vi "rpr -- read segment files.vi"(0 "9w folder path":path=path "C:/data/RUS/Experiment/ProbeTest/Probe10/YBCO_5/sweep2/9w", 2 "segment index":i32=2, 5 "buttons":bool[](array[boolean])=[TRUE, TRUE, TRUE, TRUE, TRUE, TRUE, TRUE, TRUE, TRUE, TRUE, TRUE, TRUE, TRUE, TRUE, TRUE, TRUE, TRUE, TRUE, TRUE, TRUE, TRUE, TRUE, TRUE, TRUE, TRUE, TRUE, TRUE, TRUE, TRUE], 6 "what":T2(ring)=enum."norm. attenuation", 8 "averaging window":i32=5, 10 "min T":dbl=nan, 12 "max T":dbl=nan) -> (9 "# of peaks":i32, 11 "# of temperatures":i32, 13 "K per min":dbl, 14 "peaks":i32[](array[numeric]), 16 "temperature points OUT":dbl[](array[numeric]), 17 "all peaks":i32[](array[numeric]), 18 "all unfiltered":T3(array[cluster]), 19 "Array":dbl[][](array[numeric]))   [LabVIEW 2014]
uses:
  segment file kind.ctl
  tale of three indices.vi
  Q -- check range -- i -- integer.vi
  linear interpolation - real.vi
  line -- complex.vi
  <vilib>/Analysis/baseanly.llb/A x B.vi
  <vilib>/Analysis/baseanly.llb/Real A x B.vi
  Q -- check range -- i -- real.vi
  command stack.vi
  tale of three indices -- check state.vi
  Q - not nan -- integer.vi
  Q - not nan -- real.vi
  <vilib>/Utility/file.llb/Read From Spreadsheet File.vi
  <vilib>/Utility/file.llb/Read From Spreadsheet File (string).vi
  <vilib>/Analysis/Matrix/Numeric/Conversions/Array To Matrix.vi
  <vilib>/Analysis/Matrix/Numeric/Conversions/Array To Matrix - RA2.vi
  <vilib>/Analysis/baseanly.llb/Inverse Matrix.vi
  <vilib>/Analysis/baseanly.llb/Real Inverse Matrix.vi
  <vilib>/regexp/Match Regular Expression.xnode
  <vilib>/Analysis/NI_AALBase.lvlib
panel:
  in  "segment file kind":T1
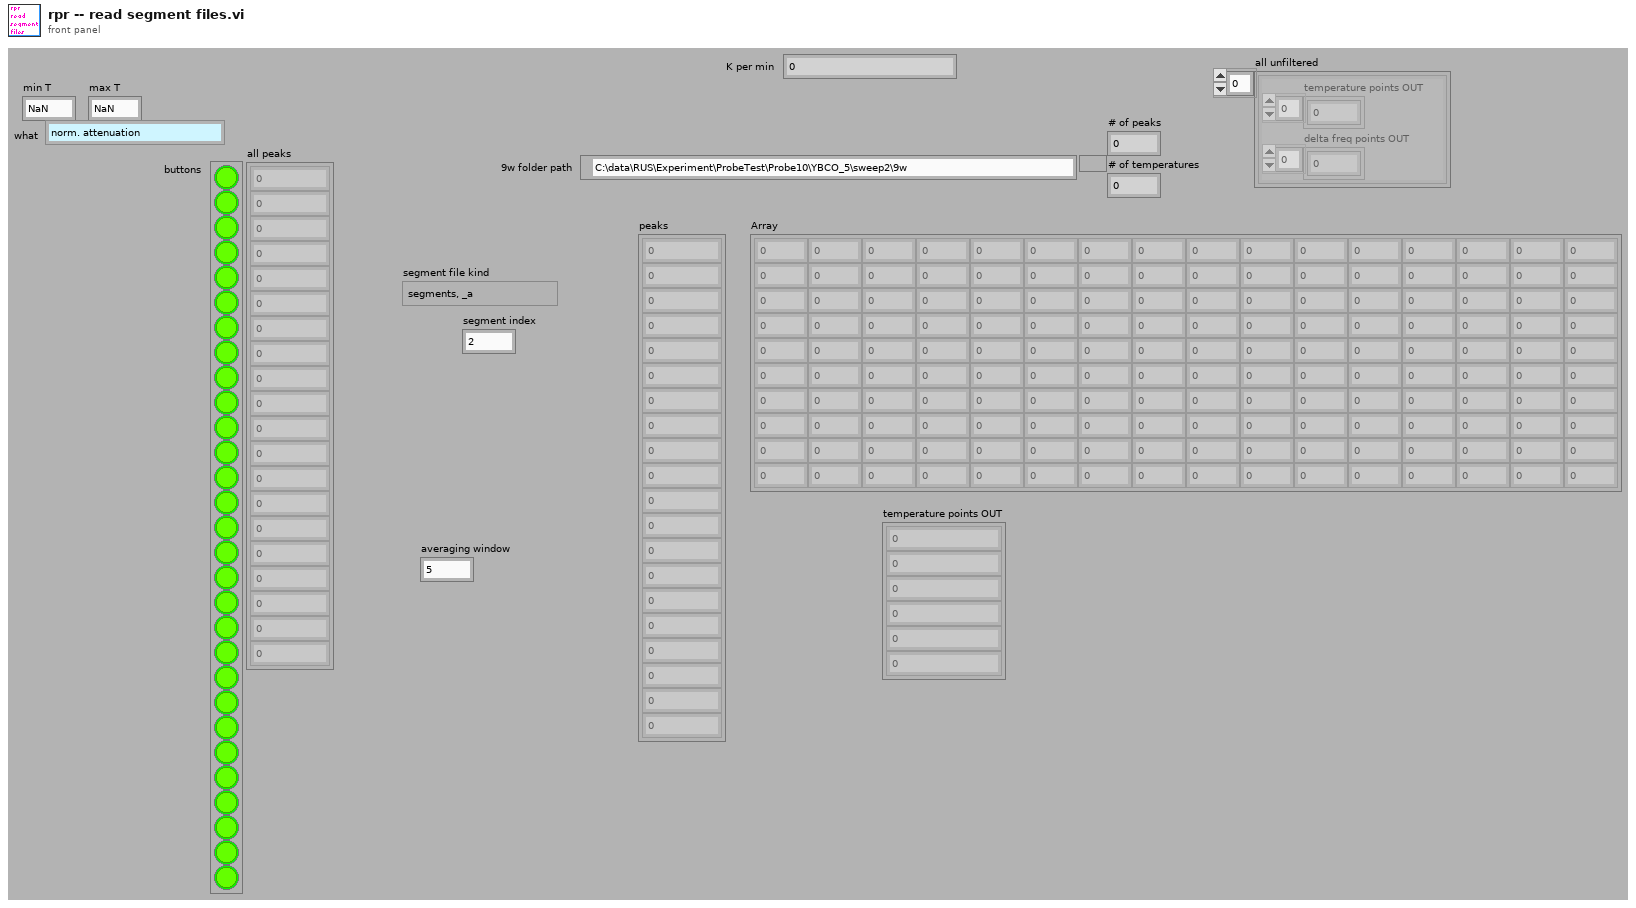
[diagram p1: front panel]
types:
  T1 = typedef "segment file kind.ctl" = enum16{"segments, _a", "monitor, _m", "other"}
  T2 = enum16{"frequency", "attenuation", "deltafreq", "Vardeltafreq", "log 1/Q", "1/Q", "norm. attenuation", "log gamma", "VarDeltaFreq div f"}
  T3 = cluster{"temperature points OUT":dbl[], "delta freq points OUT":dbl[]}[]
  T4 = cluster{"temperature points OUT":dbl[], "z out":dbl[]}
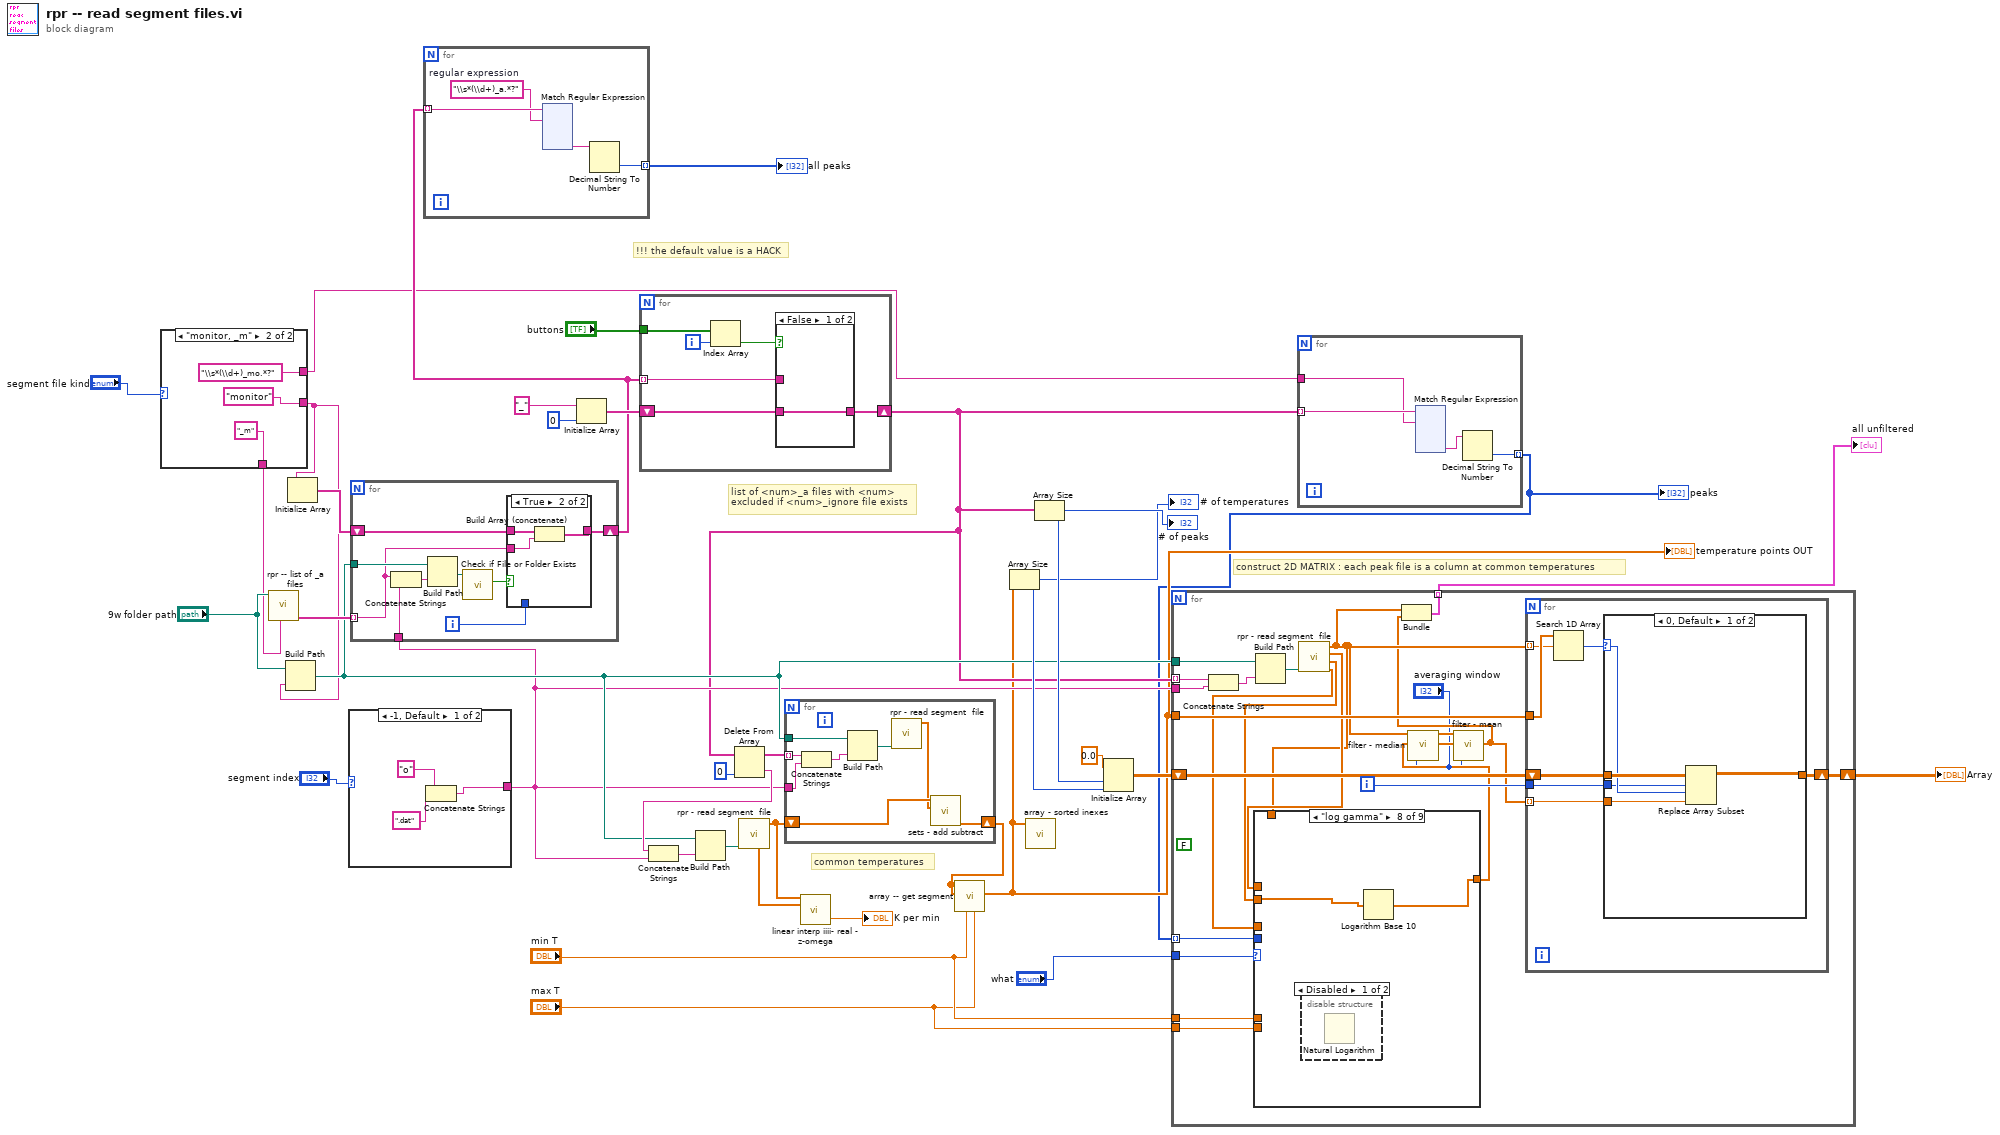
[diagram p0: block diagram]
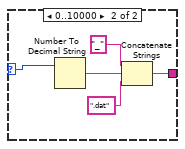
[diagram p2: hidden frame]
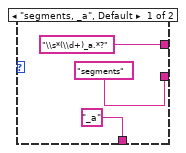
[diagram p3: hidden frame]
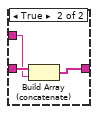
[diagram p4: hidden frame]
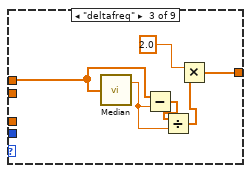
[diagram p8: hidden frame]
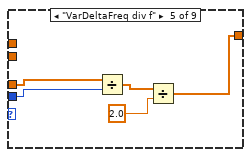
[diagram p10: hidden frame]
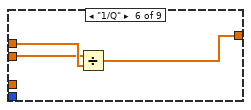
[diagram p11: hidden frame]
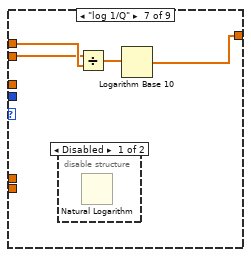
[diagram p12: hidden frame]
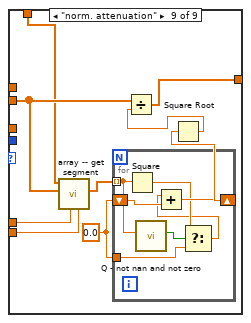
[diagram p15: hidden frame]
diagram:
  # "!!! the default value is a HACK"
  # "list of <num>_a files with <num> \nexcluded if <num>_ignore file exists"
  # "construct 2D MATRIX : each peak file is a column at common temperatures"
  # "common temperatures"
  n1 = case shown="\"monitor, _m\"" "segment file kind" {
    tunnel: ["segments" ("string") "monitor" ("string")] -> w7
    tunnel: ["_a" ("string") "_m" ("string")] -> w6
    tunnel: ["\\s*(\\d+)_a.*?" ("regular expression") "\\s*(\\d+)_mo.*?" ("regular expression")] -> w5
    frame "segments, _a", Default {
    }
    frame "monitor, _m" {
    }
  }
  n2 = call "rpr -- list of _a files.vi"("suffix"=w6, "9w folder path"="9w folder path") -> ("Array"=w28:string[])  [unwired: 9 in]
  n3 = Build Path(base path="9w folder path", name or relative path=w7) -> (appended path=w26:path)
  n4 = Initialize Array(w7) -> (w16:string[])  [unwired: 1 in]
  n5 = case shown="-1, Default" "segment index" {
    selector: "segment index" -> [_ w47]
    tunnel: [w45 w48] -> w25
    frame -1, Default {
      n6 = Concatenate Strings("o" ("string"), ".dat" ("string")) -> (w45:string)
    }
    frame 0..10000 {
      n7 = Number To Decimal String(number=w47) -> (decimal integer string=w51:string)  [unwired: 1 in]
      n8 = Concatenate Strings("_" ("string"), w51, ".dat" ("string")) -> (w48:string)
    }
  }
  n9 = for {
    tunnel: w26 -> [w59]
    tunnel: w28 -> [w52] mode=indexing
    tunnel: w25 -> [w58]
    shift-right: [w55] -> w18
    shift-left: w16 -> [w56]
    i -> [w54]
    n10 = Concatenate Strings(w52, w58) -> (w60:string)
    n11 = Build Path(base path=w59, name or relative path=w60) -> (appended path=w57:path)
    n12 = call <vilib>:"Check if File or Folder Exists.vi"("path"=w57) -> ("file or folder exists?"=w53:bool)  [unwired: 8 in, 2 out]
    n13 = case shown="True" w53 {
      tunnel: w56 -> [w61 w64]
      tunnel: [w61 w62] -> w55
      tunnel: w54 -> [_ _]
      tunnel: w52 -> [_ w63]
      frame False {
      }
      frame True {
        n14 = Build Array (concatenate)(w64, w63) -> (w62:string[])
      }
    }
  }
  n15 = for {
    tunnel: w18 -> [w68] mode=indexing
    tunnel: [w65] -> w22 mode=indexing
    w67 = "\\s*(\\d+)_a.*?"  # regular expression
    n16 = xnode "Match Regular Expression"("input string"=w68, "regular expression"=w67) -> ("submatch 1"=w66:string)  [unwired: 4 in, 5 out]
    n17 = Decimal String To Number(string=w66) -> (number=w65:i32)  [unwired: 2 in, 1 out]
  }
  "all peaks" <- w22
  n18 = Initialize Array("_" ("string"), 0 ("index")) -> (w19:string[])
  n19 = for {
    tunnel: w18 -> [w182] mode=indexing
    tunnel: "buttons" -> [w187]
    shift-right: [w183] -> w17
    shift-left: w19 -> [w184]
    i -> [w186]
    n20 = Index Array(array=w187, index=w186) -> (element=w185:bool)
    n21 = case shown="False" w185 {
      tunnel: w184 -> [w188 w191]
      tunnel: [w188 w190] -> w183
      tunnel: w182 -> [_ w189]
      frame False {
      }
      frame True {
        n22 = Build Array (concatenate)(w191, w189) -> (w190:string[])
      }
    }
  }
  n23 = Delete From Array(array=w17, index=0) -> (deleted portion=w33:string, array with subset deleted=w36:string[])  [unwired: 1 in]
  n24 = Concatenate Strings(w33, w25) -> (w34:string)
  n25 = Build Path(base path=w26, name or relative path=w34) -> (appended path=w35:path)
  n26 = call "rpr - read segment  file.vi"("file path"=w35) -> ("temperature points OUT"=w3:dbl[], "time (min) points out"=w2:dbl[])  [unwired: 6 in, 3 out]
  n27 = for {
    tunnel: w36 -> [w199] mode=indexing
    tunnel: w26 -> [w196]
    shift-right: [w193] -> w14
    shift-left: w3 -> [w195]
    tunnel: w25 -> [w192]
    n28 = Concatenate Strings(w199, w192) -> (w197:string)
    n29 = Build Path(base path=w196, name or relative path=w197) -> (appended path=w198:path)
    n30 = call "rpr - read segment  file.vi"("file path"=w198) -> ("temperature points OUT"=w194:dbl[])  [unwired: 6 in, 4 out]
    n31 = call "sets - add subtract.vi"("array 2"=w194, "array 1"=w195) -> ("common array"=w193:dbl[])  [unwired: 8 in, 1 out]
  }
  n32 = call "linear interp iiii- real - z-omega.vi"("z"=w3, "omega"=w2) -> ("slope"=→"K per min":dbl)  [unwired: 4 in, 9 out]
  n33 = call "array -- get segment.vi"("max T"="max T", "min T"="min T", "other points"=w14, "temperature points"=w14) -> ("other segment"=w13:dbl[])  [unwired: 7 in]
  "temperature points OUT" <- w13
  n34 = Array Size(array=w13) -> (size(s)=w29:i32)
  "# of temperatures" <- w29
  n35 = call "array - sorted inexes.vi"("x"=w13) -> ()  [unwired: 9 in, 2 out]
  n36 = Array Size(array=w17) -> (size(s)=w32:i32)
  "# of peaks" <- w32
  n37 = Initialize Array(0.0 ("element"), w32, w29) -> (w31:dbl[][])
  n38 = for {
    tunnel: w17 -> [w203] mode=indexing
    tunnel: [w201] -> w10 mode=indexing
    tunnel: w5 -> [w200]
    n39 = xnode "Match Regular Expression"("input string"=w203, "regular expression"=w200) -> ("submatch 1"=w202:string)  [unwired: 4 in, 5 out]
    n40 = Decimal String To Number(string=w202) -> (number=w201:i32)  [unwired: 2 in, 1 out]
  }
  "peaks" <- w10
  n41 = for {
    tunnel: w26 -> [w337]
    tunnel: w17 -> [w336] mode=indexing
    tunnel: w13 -> [w335]
    shift-right: [w333] -> w24
    shift-left: w31 -> [w334]
    tunnel: w25 -> [w331]
    tunnel: "what" -> [w330]
    tunnel: [w326] -> w15 mode=indexing
    tunnel: "min T" -> [w325]
    tunnel: "max T" -> [w324]
    tunnel: w10 -> [w323] mode=indexing
    i -> [w332]
    (unwired) FALSE
    n42 = Concatenate Strings(w336, w331) -> (w338:string)
    n43 = Build Path(base path=w337, name or relative path=w338) -> (appended path=w339:path)
    n44 = call "rpr - read segment  file.vi"("file path"=w339) -> ("delta freq points OUT"=w327:dbl[], "attenuation points OUT"=w328:dbl[], "frequency points OUT"=w329:dbl[], "temperature points OUT"=w322:dbl[])  [unwired: 6 in, 1 out]
    n45 = case shown="\"log gamma\"" w330 {
      tunnel: w329 -> [w340 _ w346 _ _ w356 w360 _ _]
      tunnel: [w340 w341 w342 w348 w349 w355 w357 w362 w371] -> w321
      tunnel: w328 -> [_ w341 _ _ _ w354 w359 w361 w370]
      tunnel: w327 -> [_ _ _ w348 w353 _ _ _ _]
      tunnel: w322 -> [_ _ _ _ _ _ _ _ w369]
      tunnel: w325 -> [_ _ _ _ _ _ _ _ w368]
      tunnel: w324 -> [_ _ _ _ _ _ _ _ w367]
      tunnel: w323 -> [_ _ _ _ w352 _ _ _ _]
      frame "frequency", Default {
      }
      frame "attenuation" {
      }
      frame "deltafreq" {
        n46 = call <vilib>:"Median.vi"("X"=w346) -> ("median"=w345:dbl)  [unwired: 1 out]
        n47 = Subtract(x=w346, y=w345) -> (x-y=w347:dbl[])
        n48 = Divide(x=w347, y=w345) -> (x/y=w344:dbl[])
        n49 = Multiply(x=2.0 ("element"), y=w344) -> (x*y=w342:dbl[])
      }
      frame "Vardeltafreq" {
      }
      frame "VarDeltaFreq div f" {
        n50 = Divide(x=w353, y=w352) -> (x/y=w351:dbl[])
        n51 = Divide(x=w351, y=2.0 ("element")) -> (x/y=w349:dbl[])
      }
      frame "1/Q" {
        n52 = Divide(x=w354, y=w356) -> (x/y=w355:dbl[])
      }
      frame "log 1/Q" {
        n53 = disable-structure shown="Disabled" {
          frame Disabled {
            n54 = Natural Logarithm() -> ()  [unwired: 1 in, 1 out]
          }
          frame Enabled {
          }
        }
        n55 = Divide(x=w359, y=w360) -> (x/y=w358:dbl[])
        n56 = Logarithm Base 10(1:w358) -> (0:w357:dbl[])
      }
      frame "log gamma" {
        n57 = disable-structure shown="Disabled" {
          frame Disabled {
            n58 = Natural Logarithm() -> ()  [unwired: 1 in, 1 out]
          }
          frame Enabled {
          }
        }
        n59 = Logarithm Base 10(1:w361) -> (0:w362:dbl[])
      }
      frame "norm. attenuation" {
        w363 = 0.0
        n60 = call "array -- get segment.vi"("max T"=w367, "min T"=w368, "other points"=w370, "temperature points"=w369) -> ("other segment"=w366:dbl[])  [unwired: 7 in]
        n61 = for {
          shift-right: [w378] -> w365
          shift-left: w363 -> [w377]
          tunnel: w366 -> [w376] mode=indexing
          tunnel: w363 -> [w373]
          n62 = Square(x=w376) -> (x^2=w374:dbl)
          n63 = call "Q - not nan and not zero.vi"("Numeric"=w376) -> ("Boolean"=w375:bool)  [unwired: 10 in]
          n64 = Select(t=w374, s=w375, f=w373) -> (s? t:f=w372:dbl)
          n65 = Add(x=w372, y=w377) -> (x+y=w378:dbl)
        }
        n66 = Square Root(x=w365) -> (sqrt(x)=w364:dbl)
        n67 = Divide(x=w370, y=w364) -> (x/y=w371:dbl[])
      }
    }
    n68 = call "filter - median.vi"("omega  in"=w322, "z in"=w321, "window"="averaging window") -> ("omega out"=w320:dbl[], "z out"=w319:dbl[])  [unwired: 14 in, 1 out]
    n69 = call "filter - mean.vi"("omega  in"=w320, "z in"=w319, "window"="averaging window") -> ("z out"=w318:dbl[])  [unwired: 13 in, 3 out]
    n70 = Bundle("temperature points OUT"=w322, "z out"=w318) -> (w326:T4)  [unwired: 1 in]
    n71 = for {
      tunnel: w322 -> [w381] mode=indexing
      tunnel: w335 -> [w384]
      shift-right: [w382] -> w333
      shift-left: w334 -> [w383]
      tunnel: w332 -> [w380]
      tunnel: w318 -> [w379] mode=indexing
      n72 = Search 1D Array(1D array=w384, element=w381) -> (index of element=w385:i32)  [unwired: 1 in]
      n73 = case shown="0, Default" w385 {
        selector: w385 -> [w387 _]
        tunnel: w383 -> [w390 w391]
        tunnel: [w389 w391] -> w382
        tunnel: w379 -> [w388 _]
        tunnel: w380 -> [w386 _]
        frame 0, Default {
          n74 = Replace Array Subset(array=w390, new element=w388, index (row)=w386, index (col)=w387) -> (w389:dbl[][])
        }
        frame -1 {
        }
      }
    }
  }
  "Array" <- w24
  "all unfiltered" <- w15
